vi "CMN_Struct2Str.vi"(8 "separator":string="=", 9 "Controls text In":string, 10 "Cluster Ref":refnum<vi>) -> (2 "Controls Text":string, 3 "Controls Array":string[][](table))   [LabVIEW 2016]
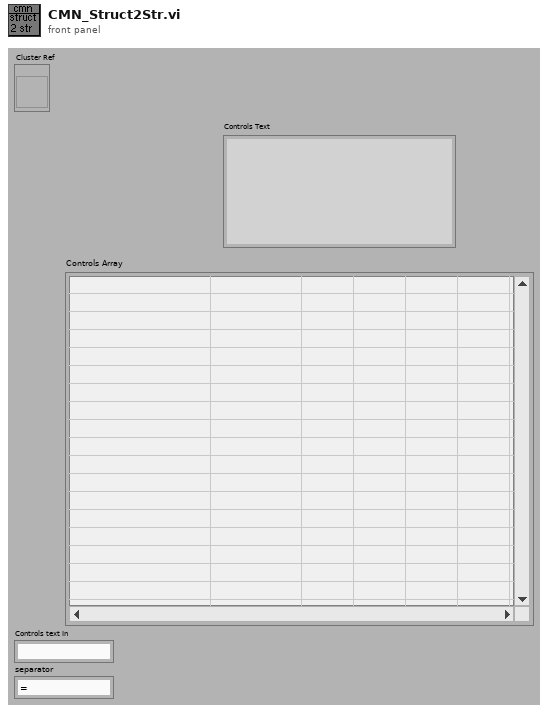
[diagram p1: front panel]
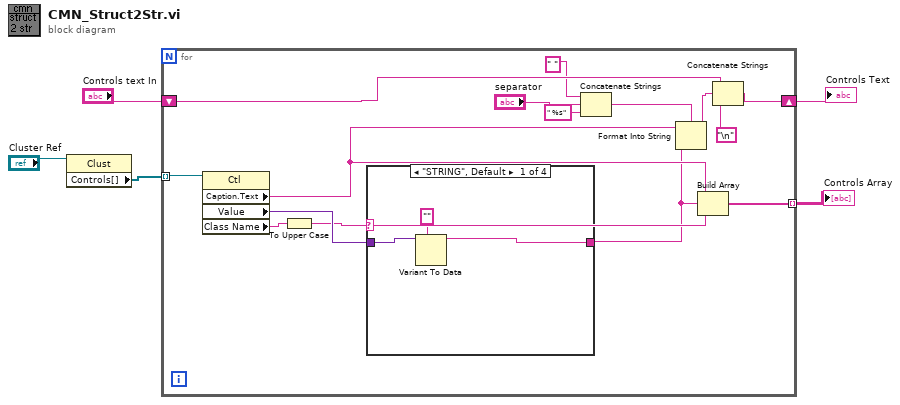
[diagram p0: block diagram]
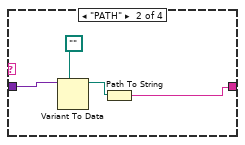
[diagram p2: hidden frame]
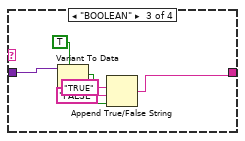
[diagram p3: hidden frame]
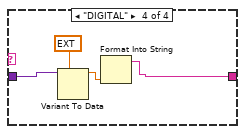
[diagram p4: hidden frame]
diagram:
  n1 = property class="Clust"(reference="Cluster Ref") -> ("Controls[]"=w4:refnum<vi>[])  [unwired: 1 in, 2 out]
  n2 = for {
    tunnel: w4 -> [w6] mode=indexing
    tunnel: [w18] -> w3 mode=indexing
    shift-right: [w16] -> w2
    shift-left: "Controls text In" -> [w13]
    n3 = property class="Ctl"(reference=w6) -> ("Caption.Text"=w17:string, "Value"=w19:variant, "Class Name"=w20:string)  [unwired: 1 in, 2 out]
    n4 = To Upper Case(1:w20) -> (0:w12:string)
    n5 = case shown="\"STRING\", Default" w12 {
      tunnel: w19 -> [w23 w27 w33 w37]
      tunnel: [w21 w24 w28 w34] -> w11
      frame "STRING", Default {
        n6 = Variant To Data(type="", Variant=w23) -> (data=w21:string)  [unwired: 1 in, 1 out]
      }
      frame "PATH" {
        n7 = Variant To Data(type=path "", Variant=w27) -> (data=w25:path)  [unwired: 1 in, 1 out]
        n8 = Path To String(path=w25) -> (string=w24:string)
      }
      frame "BOOLEAN" {
        n9 = Variant To Data(type=TRUE, Variant=w33) -> (data=w31:bool)  [unwired: 1 in, 1 out]
        n10 = Append True/False String(1:w31, 2:"FALSE" ("false string"), 3:"TRUE" ("true string")) -> (0:w28:string)  [unwired: 1 out]
      }
      frame "DIGITAL" {
        n11 = Variant To Data(type=ext 0.0, Variant=w37) -> (data=w35:ext)  [unwired: 1 in, 1 out]
        n12 = Format Into String(w35) -> (resulting string=w34:string)  [unwired: 3 in, 1 out]
      }
    }
    n13 = Concatenate Strings(" ", "separator", " %s" ("string")) -> (w9:string)
    n14 = Format Into String(format string=w9, initial string=w17, w11) -> (resulting string=w15:string)  [unwired: 1 in, 1 out]
    n15 = Build Array(w17, w11, w12) -> (w18:string[])
    n16 = Concatenate Strings(w13, w15, "\n") -> (w16:string)
  }
  "Controls Array" <- w3
  "Controls Text" <- w2
